vi "get boat location.vi"(2 "Tug":string="L", 3 "Nav String":string="$,G,43,13,230,P,10,20,120,T,10,10,330,L,14,36,110,A,3,5,B,7,8,C,16,20,D,-1,-1,S,08,12,234\r") -> (0 "Valid ?":bool, 1 "Tug Nav Data":T1)   [LabVIEW 2013]
doc: "This VI gets the location for the Tug specified along with the time data for the data. The output cluster has which boat it is, x, y, and angle, in that order."
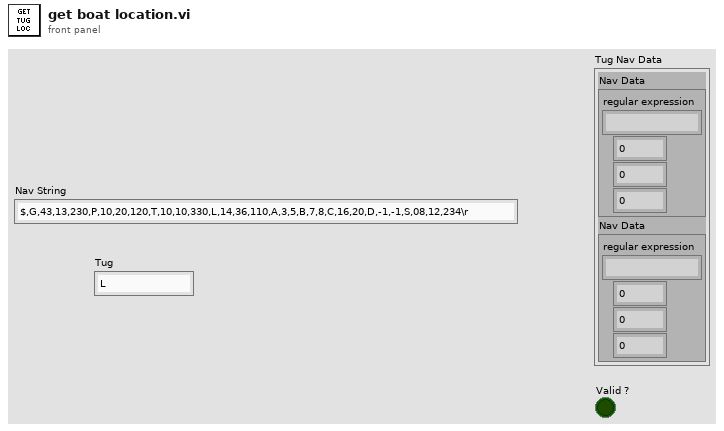
[diagram p1: front panel]
types:
  T1 = cluster{"Nav Data":cluster{"regular expression":string, i32, i32, i32}, "Nav Data":cluster{"regular expression":string, i32, i32, i32}}
  T2 = cluster{"regular expression":string, i32, i32, i32}
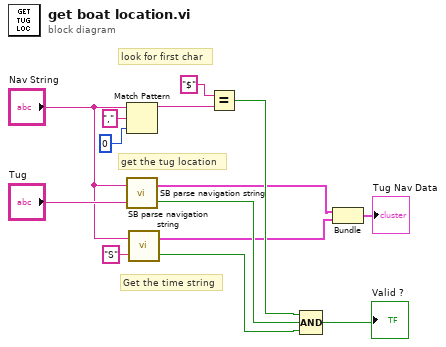
[diagram p0: block diagram]
diagram:
  # "get the tug location"
  # "Get the time string"
  # "look for first char"
  n1 = Match Pattern(string="Nav String", regular expression=",", offset (0)=0) -> (before substring=w13:string)  [unwired: 3 out]
  n2 = call "SB parse navigation string.vi"("Header"="Tug", "Nav String"="Nav String") -> ("Valid?"=w7:bool, "Nav Data"=w4:T2)
  n3 = call "SB parse navigation string.vi"("Header"="S", "Nav String"="Nav String") -> ("Valid?"=w6:bool, "Nav Data"=w3:T2)
  n4 = Equal?(x="$", y=w13) -> (x = y?=w8:bool)
  n5 = Compound Arithmetic op=AND(w8, w7, w6) -> (→"Valid ?":bool)
  n6 = Bundle("Nav Data"=w4, "Nav Data"=w3) -> (→"Tug Nav Data":T1)  [unwired: 1 in]
